vi "ProgramControlProgramStatus.vi"(0 "Front Panel Controls in":T2, 5 "Program State":T1) -> (14 "Front Panel Controls out":T2)   [LabVIEW 2019, in "Universal Robot.lvclass"]
uses:
  Universal Robot.lvclass
  ProgramControlFPControls.ctl
  ProgramState.ctl
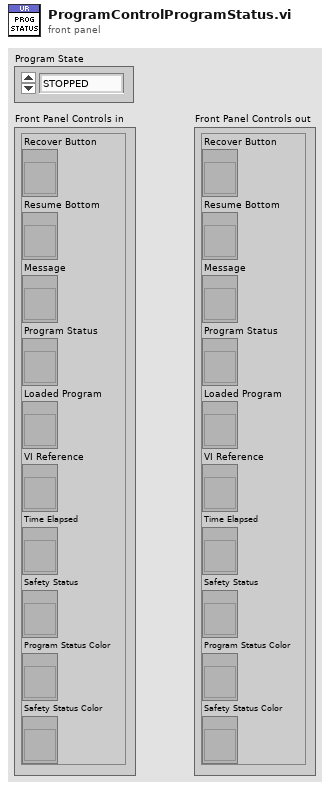
[diagram p1: front panel]
types:
  T1 = typedef "Universal Robot.lvclass/ProgramState.ctl" = enum16{"STOPPED", "PLAYING", "PAUSE"}
  T2 = typedef "Universal Robot.lvclass/ProgramControlFPControls.ctl" = cluster{"Recover Button":refnum<vi>, "Resume Bottom":refnum<vi>, "Message":refnum<vi>, "Program Status":refnum<vi>, "Loaded Program":refnum<vi>, "VI Reference":refnum<vi>, "Time Elapsed":refnum<vi>, "Safety Status":refnum<vi>, "Program Status Color":refnum<vi>, "Safety Status Color":refnum<vi>}
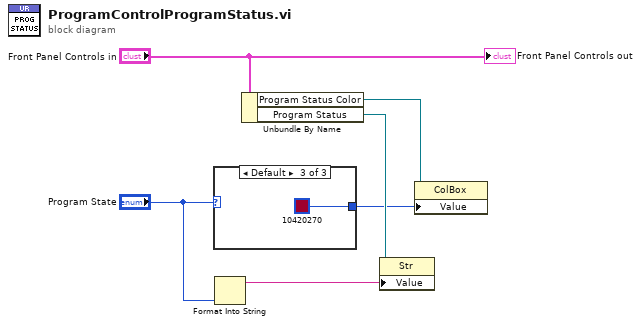
[diagram p0: block diagram]
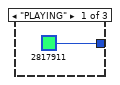
[diagram p2: hidden frame]
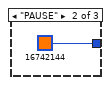
[diagram p3: hidden frame]
diagram:
  n1 = case shown="Default" "Program State" {
    tunnel: [u32 2817911 u32 16742144 u32 10420270] -> w2
    frame "PLAYING" {
    }
    frame "PAUSE" {
    }
    frame Default {
    }
  }
  n2 = Format Into String("Program State") -> (resulting string=w4:string)  [unwired: 3 in, 1 out]
  n3 = Unbundle By Name("Front Panel Controls in") -> ("Program Status Color"=w3:refnum<vi>, "Program Status"=w5:refnum<vi>)
  n4 = property class="Str"(reference=w5, "Value"=w4) -> ()  [unwired: 1 in, 2 out]
  n5 = property class="ColBox"(reference=w3, "Value"=w2) -> ()  [unwired: 1 in, 2 out]
  "Front Panel Controls out" <- "Front Panel Controls in"
